vi "ArmCurls.vi"(9 "Actual Shoulder Angle (deg)":dbl, 10 "Arm Speed":dbl, 11 "shoulder speed (deg/s)":dbl) -> ()   [LabVIEW 2018]
uses:
  <vilib>/Rock Robotics/Network Tables/NT Write Number.vi
panel:
  out "Elbow Speed 2":dbl
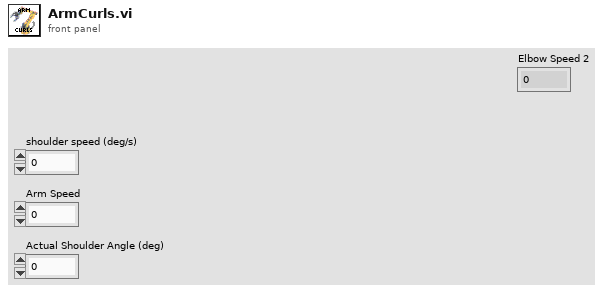
[diagram p1: front panel]
types:
  T1 = typedef "WPI_MotorControlDeviceRef.ctl" = cluster{"DeviceStatus":errorcluster, "Type":T2, "PWM":cluster{"PWM Channel":T3, "DeadBand":T4}, "CAN":cluster{"Device Number":u8, "SetOutput VI Ref":variant, "GetOutput VI Ref":variant, "Enable VI Ref":variant, "Disable VI Ref":variant, "Data":variant}, "Invert":bool, "DIO PWM":cluster{"PWM \"Enable\" Channel":T3, "DIOChannel":T5, "PWM Rate":dbl}}
  T2 = typedef "WPI_MotorControlType.ctl" = enum16{"PWM", "CAN", "DIO PWM"}
  T3 = typedef "FPGA_DIOPWMChannel.ctl" = enum8{"PWM 0", "PWM 1", "PWM 2", "PWM 3", "PWM 4", "PWM 5", "PWM 6", "PWM 7", "PWM 8", "PWM 9", "PWM MXP 0", "PWM MXP 1", "PWM MXP 2", "PWM MXP 3", "PWM MXP 4", "PWM MXP 5", "PWM MXP 6", "PWM MXP 7", "PWM MXP 8", "PWM MXP 9", "Invalid"}
  T4 = typedef "WPI_PWMDeadband.ctl" = cluster{"Name":string, "maxPositivePwm":i32, "minPositivePwm":i32, "centerPwm":i32, "maxNegativePwm":i32, "minNegativePwm":i32, "angularRange":u16}
  T5 = typedef "FPGA_DIOChannel.ctl" = enum8{"DIO 0", "DIO 1", "DIO 2", "DIO 3", "DIO 4", "DIO 5", "DIO 6", "DIO 7", "DIO 8", "DIO 9", "DIO MXP 0", "DIO MXP 1", "DIO MXP 2", "DIO MXP 3", "DIO MXP 4", "DIO MXP 5", "DIO MXP 6", "DIO MXP 7", "DIO MXP 8", "DIO MXP 9", "DIO MXP 10", "DIO MXP 11", "DIO MXP 12", "DIO MXP 13", "DIO MXP 14", "DIO MXP 15", "SPI Port CS1", "SPI Port CS2", "SPI Port CS3", "SPI Port MISO", "SPI Port MOSI", "Invalid"}
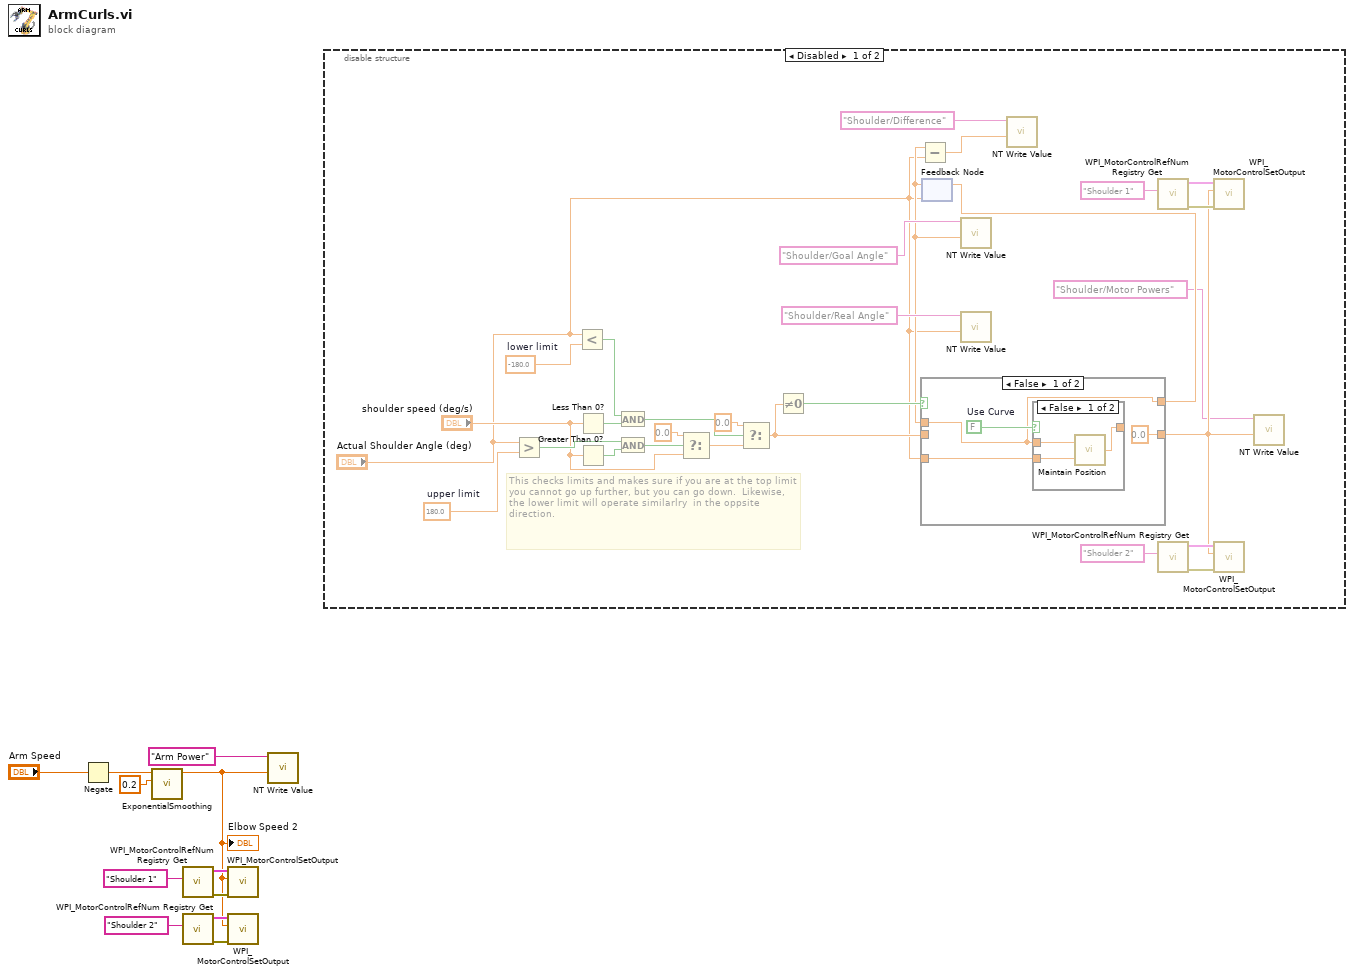
[diagram p0: block diagram]
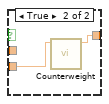
[diagram p2: hidden frame]
diagram:
  n1 = Negate(x="Arm Speed") -> (-x=w5:dbl)
  n2 = call "ExponentialSmoothing.vi"("Smoothing Factor"=0.2, "Value"=w5) -> ("Smooth Value"=w1:dbl)  [unwired: 9 in]
  "Elbow Speed 2" <- w1
  n3 = call <vilib>:"WPI_MotorControlRefNum Registry Get.vi"("refnum name"="Shoulder 1") -> ("error out"=w9:errorcluster, "MotorControlDevRef"=w10:T1)  [unwired: 9 in]
  n4 = call <vilib>:"WPI_MotorControlRefNum Registry Get.vi"("refnum name"="Shoulder 2") -> ("error out"=w3:errorcluster, "MotorControlDevRef"=w2:T1)  [unwired: 9 in]
  n5 = call <vilib>:"WPI_MotorControlSetOutput.vi"("error in (no error)"=w9, "Output"=w1, "MotorControlDevRef"=w10) -> ()  [unwired: 6 in, 3 out]
  n6 = call <vilib>:"WPI_MotorControlSetOutput.vi"("error in (no error)"=w3, "Output"=w1, "MotorControlDevRef"=w2) -> ()  [unwired: 6 in, 3 out]
  n7 = call-poly <vilib>:"NT Write Value.vi"("Numeric"=w1, "Name"="Arm Power") -> ()  [unwired: 9 in, 1 out]
  n8 = disable-structure shown="Disabled" {
    frame Disabled {
      w28 = -180.0  # lower limit
      w37 = 180.0  # upper limit
      # "This checks limits and makes sure if you are at the top limit you cannot go up further, but you can go down.  Likewise, the lower limit will operate similarlry  in the oppsite direction."
      n9 = Greater?(x="Actual Shoulder Angle (deg)", y=w37) -> (0:w35:bool)
      n10 = Less?(x="Actual Shoulder Angle (deg)", y=w28) -> (x < y?=w30:bool)
      n11 = Less Than 0?(x="shoulder speed (deg/s)") -> (x < 0?=w29:bool)
      n12 = Greater Than 0?(x="shoulder speed (deg/s)") -> (x > 0?=w36:bool)
      n13 = And(x=w30, y=w29) -> (x .and. y?=w31:bool)
      n14 = And(x=w35, y=w36) -> (x .and. y?=w34:bool)
      n15 = Select(t=0.0 ("f"), s=w34, f="shoulder speed (deg/s)") -> (s? t:f=w27:dbl)
      n16 = Select(t=0.0 ("f"), s=w31, f=w27) -> (s? t:f=w22:dbl)
      n17 = Not Equal To 0?(x=w22) -> (x != 0?=w23:bool)
      n18 = feedback #1("Actual Shoulder Angle (deg)") -> (w15:dbl)
      n19 = Subtract(x=w15, y="Actual Shoulder Angle (deg)") -> (x-y=w13:dbl)
      n20 = case shown="False" w23 {
        tunnel: "Actual Shoulder Angle (deg)" -> [w44 w50]
        tunnel: [0.0 ("shoulder speed (deg/s)") w51] -> w18
        tunnel: w22 -> [_ w51]
        tunnel: [w42 w50] -> w20
        tunnel: w15 -> [w42 _]
        frame False {
          w43 = FALSE  # Use Curve
          n21 = case shown="False" w43 {
            tunnel: w44 -> [w46 w49]
            tunnel: [w45 w48] -> _
            tunnel: w42 -> [w47 _]
            frame False {
              n22 = call "Maintain Position.vi"("Real Angle"=w46, "Goal Angle"=w47) -> ("Output"=w45:dbl)
            }
            frame True {
              n23 = call "Counterweight.vi"("Current Angle"=w49) -> ("Current Counter Weight Power"=w48:dbl)  [unwired: 10 in]
            }
          }
        }
        frame True {
        }
      }
      n24 = feedback-in #1(w20) -> ()
      n25 = call-poly <vilib>:"NT Write Value.vi"("Numeric"=w15, "Name"="Shoulder/Goal Angle") -> ()  [unwired: 9 in, 1 out]
      n26 = call-poly <vilib>:"NT Write Value.vi"("Numeric"="Actual Shoulder Angle (deg)", "Name"="Shoulder/Real Angle") -> ()  [unwired: 9 in, 1 out]
      n27 = call-poly <vilib>:"NT Write Value.vi"("Numeric"=w13, "Name"="Shoulder/Difference") -> ()  [unwired: 9 in, 1 out]
      n28 = call <vilib>:"WPI_MotorControlRefNum Registry Get.vi"("refnum name"="Shoulder 1") -> ("error out"=w38:errorcluster, "MotorControlDevRef"=w39:T1)  [unwired: 9 in]
      n29 = call <vilib>:"WPI_MotorControlRefNum Registry Get.vi"("refnum name"="Shoulder 2") -> ("error out"=w25:errorcluster, "MotorControlDevRef"=w24:T1)  [unwired: 9 in]
      n30 = call <vilib>:"WPI_MotorControlSetOutput.vi"("error in (no error)"=w38, "Output"=w18, "MotorControlDevRef"=w39) -> ()  [unwired: 6 in, 3 out]
      n31 = call <vilib>:"WPI_MotorControlSetOutput.vi"("error in (no error)"=w25, "Output"=w18, "MotorControlDevRef"=w24) -> ()  [unwired: 6 in, 3 out]
      n32 = call-poly <vilib>:"NT Write Value.vi"("Numeric"=w18, "Name"="Shoulder/Motor Powers") -> ()  [unwired: 9 in, 1 out]
    }
    frame Enabled {
    }
  }
